vi "hmi_initialize.vi"(7 "hmi_references":T1, 8 "error in (no error)":errorcluster) -> (0 "error out":errorcluster)   [LabVIEW 2015, in "lv-interface-dom-nre.lvlib"]
uses:
  lv-interface-dom-nre.lvlib
  _controls/hmi_references.ctl
  lv-interface-sub-common/_controls/interface_selection.ctl
  lv-interface-sub-common/lv-interface-sub-common.lvlib
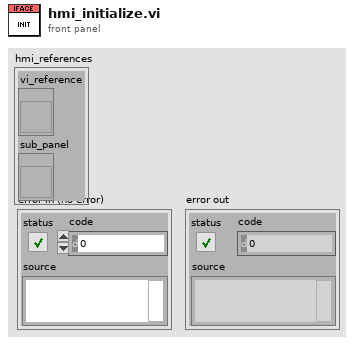
[diagram p1: front panel]
types:
  T1 = typedef "lv-interface-dom-nre.lvlib/hmi_references.ctl" = cluster{"vi_reference":refnum<vi>, "sub_panel":refnum<vi>}
  T2 = typedef "lv-interface-sub-common.lvlib/interface_selection.ctl" = enum16{"<interface>", "sub_interface_1", "sub_interface_2", "<null>"}
  T3 = enum32{"Invalid", "Standard", "Closed", "Hidden", "Minimized", "Maximized"}
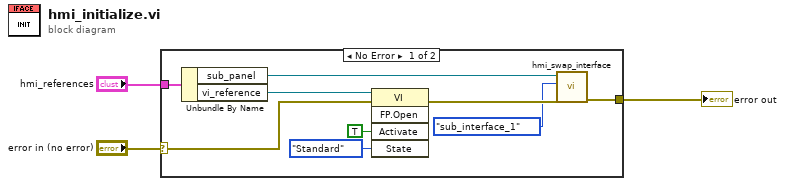
[diagram p0: block diagram]
diagram:
  n1 = case shown="No Error" "error in (no error)" {
    selector: "error in (no error)" -> [w8 w13]
    tunnel: [w5 w13] -> w2
    tunnel: "hmi_references" -> [w9 _]
    frame No Error {
      n2 = Unbundle By Name(w9) -> ("sub_panel"=w7:refnum<vi>, "vi_reference"=w12:refnum<vi>)
      n3 = invoke class="VI" method="FP.Open"(reference=w12, error in=w8, "Activate"=TRUE ("Activate?"), "State"=T3."Standard") -> (error out=w6:errorcluster)  [unwired: 1 in, 4 out]
      n4 = call "hmi_swap_interface.vi"("error in (no error)"=w6, "interface"=interface_selection."sub_interface_1", "subpanel_reference"=w7) -> ("error out"=w5:errorcluster)  [unwired: 8 in]
    }
    frame Error {
    }
  }
  "error out" <- w2
